vi "inverse_kinematics.vi"(8 "error in":errorcluster, 9 "Initial axis positions":dbl[](array[numeric])=[0.0, 0.0, 0.0, 0.0, 0.0, 0.0], 10 "Pose":T2) -> (0 "error out":errorcluster, 1 "f(minimum)":dbl, 2 "Axis positions":dbl[](array[numeric]), 4 "Error":string, 6 "number of function evaluations":i32)   [LabVIEW 2014]
uses:
  <vilib>/Analysis/Matrix/Datatypes/RealMatrix.ctl
  <vilib>/gmath/NumericalOptimization/stopping criteria.ctl
  <vilib>/gmath/NI_Gmath.lvlib
  <vilib>/gmath/NumericalOptimization/Downhill Simplex.vi
  <vilib>/Analysis/Matrix/NI_Matrix.lvlib
panel:
  in  "stopping criteria":T1={"function tolerance"=0.0001, "parameter tolerance"=0.0001, "max iterations"=100000, "max function calls"=100000, "gradient tolerance"=0.0001, "max time (sec)"=0.1}
  # "Find the inverse kinematics of the motion stage: the axis positions that generate the specified output pose."
  # "### not actually using optimization, just a simple closed form expression works better.\n\nIt doesn't seem that the tolerance criteria actually cause stopping with downhill simplex.  The optimization isn't working all that great either, converging pretty slowly and claiming not to find a minimum, even when it drives the error to zero. \n\nThere are much more efficient ways to solve inverse kinematics, but this seems to be working well enough for this use."
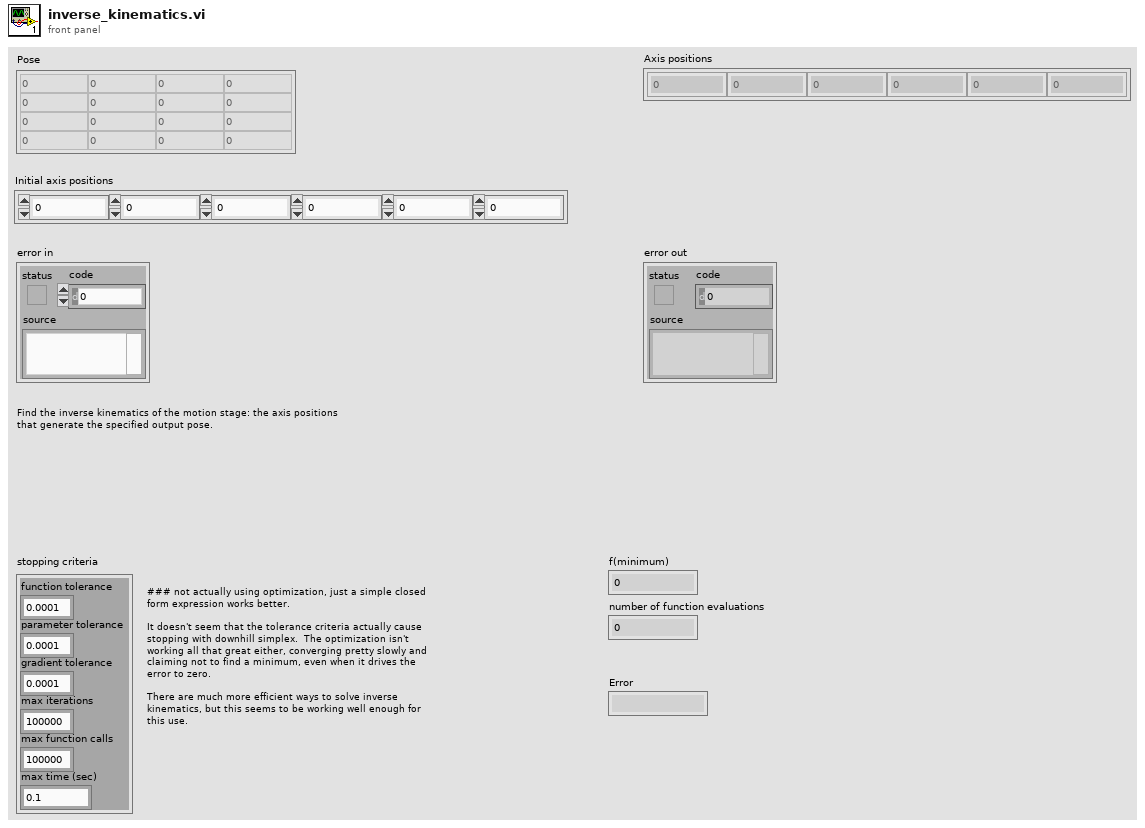
[diagram p1: front panel]
types:
  T1 = typedef "NI_Gmath.lvlib/stopping criteria.ctl" = cluster{"function tolerance":dbl, "parameter tolerance":dbl, "max iterations":i32, "max function calls":i32, "gradient tolerance":dbl, "max time (sec)":dbl}
  T2 = typedef "NI_Matrix.lvlib/RealMatrix.ctl" = dbl[][]
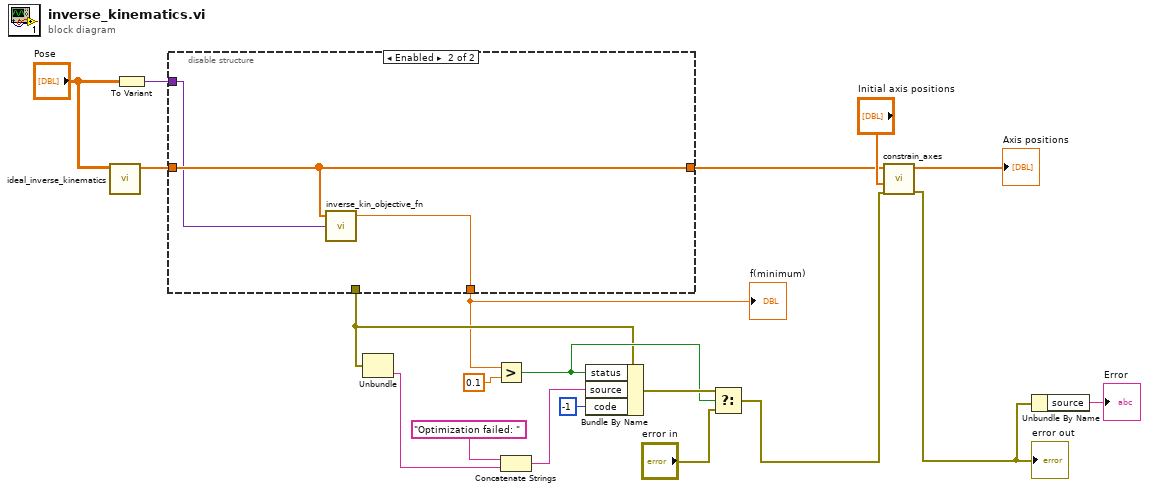
[diagram p0: block diagram]
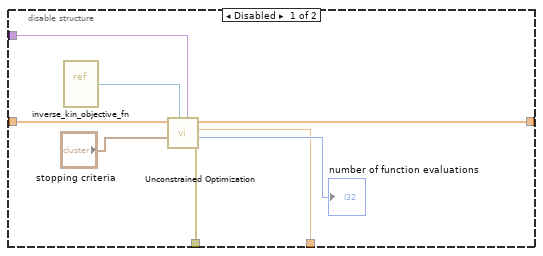
[diagram p2: hidden frame]
diagram:
  n1 = call "ideal_inverse_kinematics.vi"("Pose"="Pose") -> ("Axis positions"=w9:dbl[])  [unwired: 10 in]
  n2 = To Variant(anything="Pose") -> (Variant=w7:variant)
  n3 = disable-structure shown="Enabled" {
    disable-tunnel: [w24 w30] -> w1
    disable-tunnel: [w23 w29] -> w6
    disable-tunnel: [w22 _] -> w12
    disable-tunnel: w7 -> [w20 w28]
    disable-tunnel: w9 -> [w21 w30]
    frame Disabled {
      n4 = vi-ref "inverse_kin_objective_fn.vi"() -> (w27:refnum<vi>)
      n5 = call-poly <vilib>:"Unconstrained Optimization.vi"("function data"=w20, "objective function"=w27, "stopping criteria"="stopping criteria", "start"=w21) -> ("error out"=w22:errorcluster, "number of function evaluations"=→"number of function evaluations":i32, "f(minimum)"=w23:dbl, "minimum"=w24:dbl[])  [unwired: 4 in]
    }
    frame Enabled {
      n6 = call "inverse_kin_objective_fn.vi"("data"=w28, "X"=w30) -> ("f(X)"=w29:dbl)  [unwired: 1 in, 2 out]
    }
  }
  "f(minimum)" <- w6
  n7 = Unbundle(w12) -> ("source"=w16:string)  [unwired: 2 out]
  n8 = Greater?(x=w6, y=0.1) -> (0:w13:bool)
  n9 = Concatenate Strings("Optimization failed: " ("string"), w16) -> (w15:string)
  n10 = Bundle By Name(cluster=w12, "status"=w13, "source"=w15, "code"=-1) -> (w14:errorcluster)
  n11 = Select(t=w14, s=w13, f="error in") -> (s? t:f=w3:errorcluster)
  n12 = call "constrain_axes.vi"("error in"=w3, "Axis current positions"="Initial axis positions", "Axis positions in"=w1) -> ("error out"=w2:errorcluster, "Axis positions out"=→"Axis positions":dbl[])  [unwired: 6 in, 1 out]
  "error out" <- w2
  n13 = Unbundle By Name(w2) -> ("source"=→"Error":string)
